vi "Multicolumn listbox Helper.vi"(4 "Row to Delete":i32, 5 "Sheet Colors":T1, 6 "Visible rows":i32=16, 7 "Multicolumn Ref":refnum<vi>, 8 "Error In":errorcluster, 9 "2D Data":string[][](array[string]), 10 "Data":string[](array[string]), 11 "Action (add default)":T2=enum."Add") -> (0 "Error Out":errorcluster)   [LabVIEW 2012]
doc: "The .vi is used with a \"Multicolumn Listbox\" \n\nHow to use.\nInit:\n1.Reference to Multicolumn Listbox (this is a functional global so you only need to set it once)\n2.Set action to Init\n3.Set names on columns, last column (Status) will be added automatic (Init also sets the nummber of visible columns)\n4.Set nummber of visible rows (if you add more data then visible rows the vertical scrollbar will be visible)\n5.Colors (optional) use if you want to change colors for OK, FAIL and clear (this is a functional global so you only need to set it once)\n\nClear:\nJust set Action to Clear, no other inputs needed\n\nAdd:\nTo Add data to the listbox you need to use two inputs\n1. Status sets the color of the row and OK or FAIL in the last column (Status)\n2. Data Is an array of strings, one string for each column you have defined in Init\n3.Action Add is default so it is not necessary to set\nIf you add more lines then set in init the vertical scrollbar will be visible"
uses:
  Controls/Spreadsheet Commands.ctl
  Controls/Sheet Colors.ctl
  <vilib>/Utility/miscctls.llb/LVRowAndColumnTypeDef.ctl
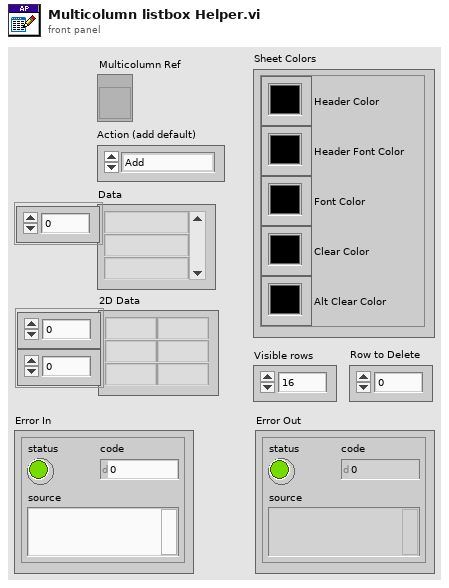
[diagram p1: front panel]
types:
  T1 = typedef "Sheet Colors.ctl" = cluster{"Header Color":u32, "Header Font Color":u32, "Font Color":u32, "Clear Color":u32, "Alt Clear Color":u32}
  T2 = typedef "Spreadsheet Commands.ctl" = enum16{"Init", "Clear", "Add", "Mass Add", "Delete Row", "Format Colors"}
  T3 = typedef "LVRowAndColumnTypeDef.ctl" = cluster{"Row":i32, "Column":i32}
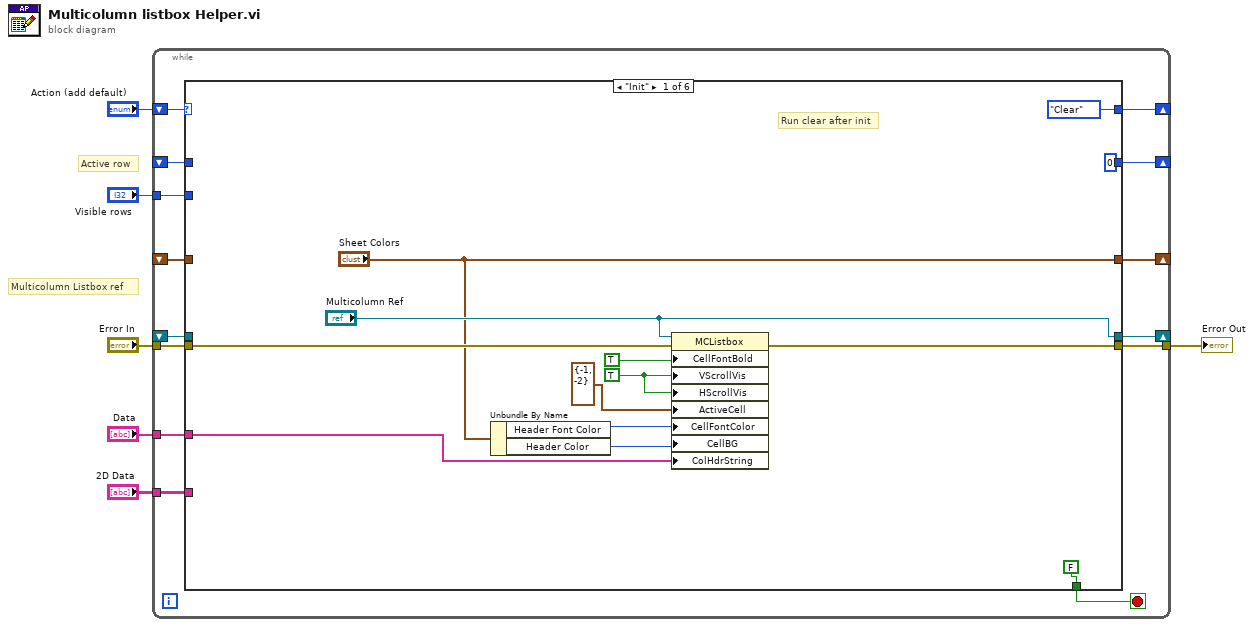
[diagram p0: block diagram]
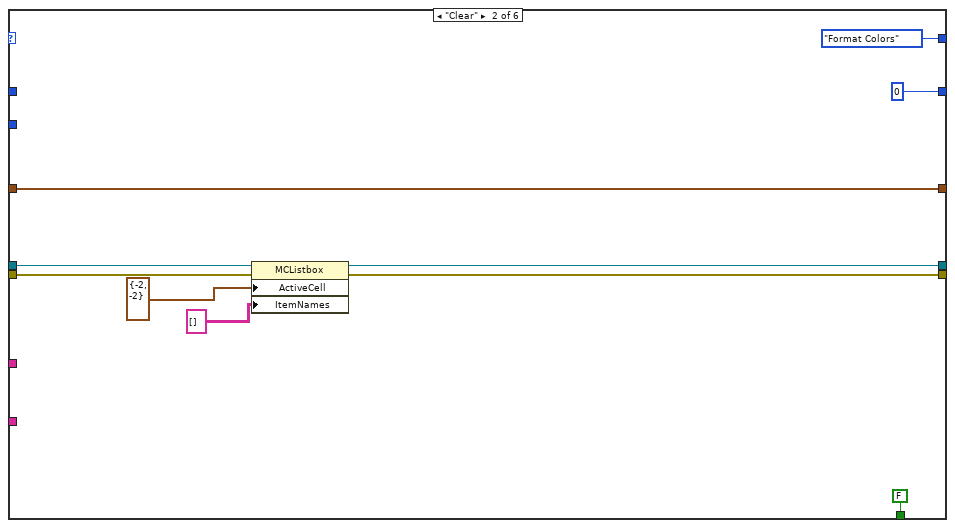
[diagram p2: hidden frame]
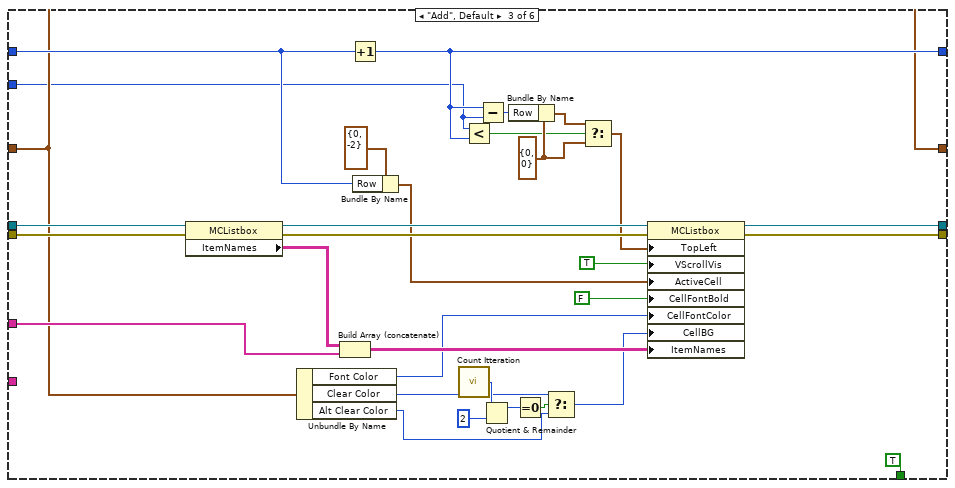
[diagram p3: hidden frame]
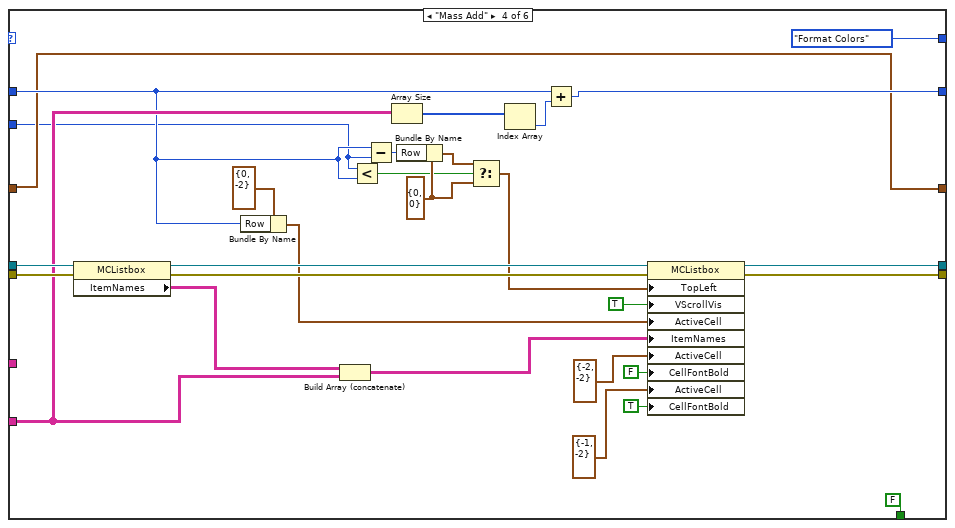
[diagram p4: hidden frame]
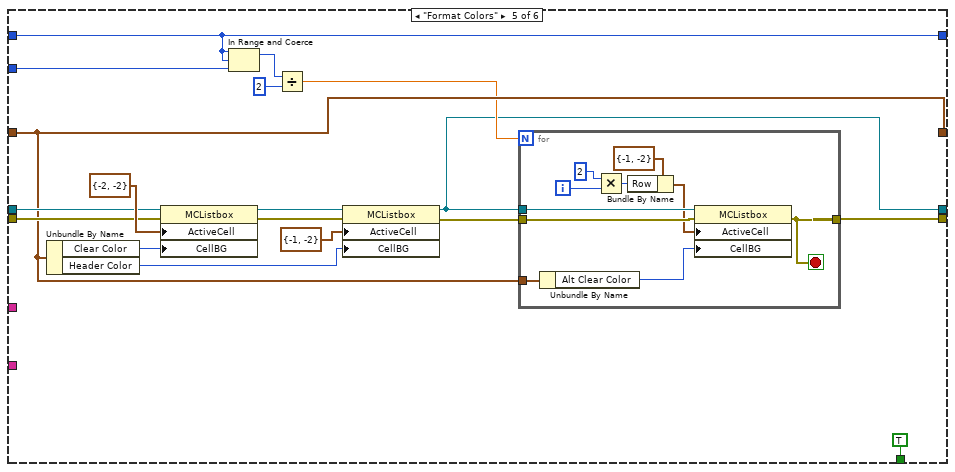
[diagram p5: hidden frame]
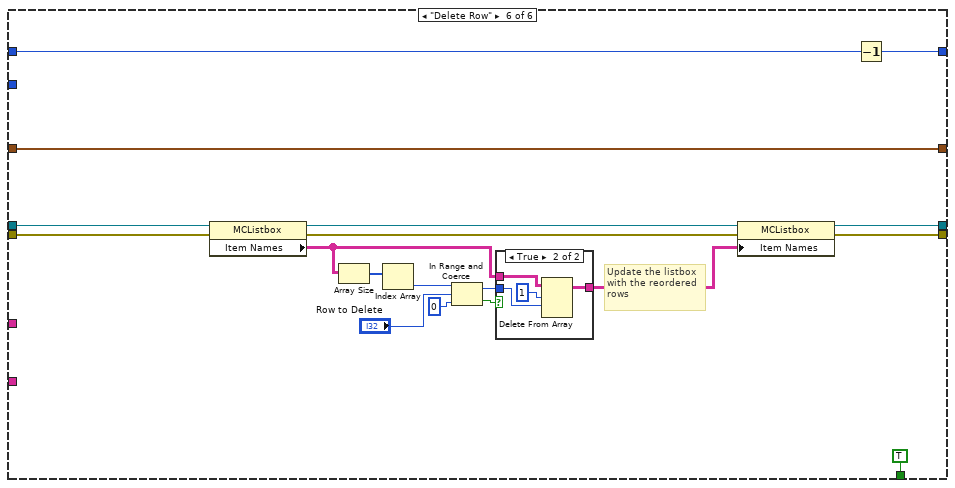
[diagram p6: hidden frame]
diagram:
  # "Active row"
  # "Multicolumn Listbox ref"
  n1 = while {
    shift-right: [w19] -> _
    shift-left: _ -> [w20]
    tunnel: "Error In" -> [w18]
    tunnel: [w17] -> w5
    shift-right: [w15] -> _
    shift-left: "Action (add default)" -> [w16]
    shift-right: [w13] -> _
    shift-left: _ -> [w12]
    tunnel: "Visible rows" -> [w11]
    tunnel: "Data" -> [w10]
    tunnel: "2D Data" -> [w9]
    shift-right: [w8] -> _
    shift-left: _ -> [w7]
    stop <- w14 stop-if-true
    n2 = case shown="\"Init\"" w16 {
      tunnel: w20 -> [_ w42 w67 w96 w118 w139]
      tunnel: ["Multicolumn Ref" w36 w63 w81 w104 w137] -> w19
      tunnel: w18 -> [w25 w41 w66 w95 w117 w140]
      tunnel: [w27 w35 w62 w93 w106 w138] -> w17
      tunnel: [Spreadsheet_Commands."Clear" ("Action (add default)") Spreadsheet_Commands."Format Colors" ("Action (add default)") _ Spreadsheet_Commands."Format Colors" ("Action (add default)") _ _] -> w15
      tunnel: [FALSE FALSE TRUE FALSE TRUE TRUE] -> w14
      tunnel: [0 ("Row") 0 ("Row") w57 w90 w108 w135] -> w13
      tunnel: w12 -> [_ _ w64 w82 w108 w136]
      tunnel: w11 -> [_ _ w44 w75 w109 _]
      tunnel: w10 -> [w26 _ w55 _ _ _]
      tunnel: w9 -> [_ _ _ w88 _ _]
      tunnel: w7 -> [_ w34 w48 w76 w110 w133]
      tunnel: ["Sheet Colors" w34 w48 w76 w110 w133] -> w8
      frame "Init" {
        w32 = TRUE
        # "Run clear after init"
        n3 = Unbundle By Name("Sheet Colors") -> ("Header Font Color"=w23:u32, "Header Color"=w24:u32)
        n4 = property class="MCListbox"(reference="Multicolumn Ref", error in=w25, "CellFontBold"=TRUE ("Active Cell:Cell Font:Bold"), "VScrollVis"=w32, "HScrollVis"=w32, "ActiveCell"=T3 {"Row"=-1, "Column"=-2} ("Active Cell:Active Cell"), "CellFontColor"=w23, "CellBG"=w24, "ColHdrString"=w26) -> (error out=w27:errorcluster)  [unwired: 1 out]
      }
      frame "Clear" {
        n5 = property class="MCListbox"(reference=w42, error in=w41, "ActiveCell"=T3 {"Row"=-2, "Column"=-2} ("Active Cell:Active Cell"), "ItemNames"=string[][] []) -> (reference out=w36:refnum<vi>, error out=w35:errorcluster)
      }
      frame "Add", Default {
        w70 = T3 {"Row"=0, "Column"=0} ("Active Cell:Active Cell")
        n6 = property class="MCListbox"(reference=w67, error in=w66) -> (reference out=w74:refnum<vi>, error out=w71:errorcluster, "ItemNames"=w60:string[][])
        n7 = Unbundle By Name(w48) -> ("Font Color"=w47:u32, "Clear Color"=w46:u32, "Alt Clear Color"=w45:u32)
        n8 = Build Array (concatenate)(w60, w55) -> (w58:string[][])
        n9 = Increment(x=w64) -> (x+1=w57:i32)
        n10 = Bundle By Name(cluster=T3 {"Row"=0, "Column"=-2} ("Active Cell:Active Cell"), "Row"=w64) -> (w61:T3)
        n11 = call "Count Itteration.vi"() -> ("Itteration"=w54:i32)  [unwired: 7 in, 1 out]
        n12 = Less?(x=w44, y=w57) -> (x < y?=w56:bool)
        n13 = Subtract(x=w57, y=w44) -> (x-y=w73:i32)
        n14 = Quotient & Remainder(x=w54, y=2) -> (x-y*floor(x/y)=w52:i32)  [unwired: 1 out]
        n15 = Bundle By Name(cluster=w70, "Row"=w73) -> (w72:T3)
        n16 = Equal To 0?(x=w52) -> (x = 0?=w51:bool)
        n17 = Select(t=w46, s=w51, f=w45) -> (s? t:f=w50:u32)
        n18 = Select(t=w72, s=w56, f=w70) -> (s? t:f=w69:T3)
        n19 = property class="MCListbox"(reference=w74, error in=w71, "TopLeft"=w69, "VScrollVis"=TRUE ("Visible Items:Vertical Scrollbar Visible"), "ActiveCell"=w61, "CellFontBold"=FALSE ("Caption.Font:Bold"), "CellFontColor"=w47, "CellBG"=w50, "ItemNames"=w58) -> (reference out=w63:refnum<vi>, error out=w62:errorcluster)
      }
      frame "Mass Add" {
        w99 = T3 {"Row"=0, "Column"=0} ("Active Cell:Active Cell")
        n20 = property class="MCListbox"(reference=w96, error in=w95) -> (reference out=w103:refnum<vi>, error out=w100:errorcluster, "ItemNames"=w91:string[][])
        n21 = Bundle By Name(cluster=T3 {"Row"=0, "Column"=-2} ("Active Cell:Active Cell"), "Row"=w82) -> (w92:T3)
        n22 = Build Array (concatenate)(w91, w88) -> (w84:string[][])
        n23 = Less?(x=w75, y=w82) -> (x < y?=w89:bool)
        n24 = Subtract(x=w82, y=w75) -> (x-y=w102:i32)
        n25 = Array Size(array=w88) -> (size(s)=w87:i32[])
        n26 = Bundle By Name(cluster=w99, "Row"=w102) -> (w101:T3)
        n27 = Select(t=w101, s=w89, f=w99) -> (s? t:f=w98:T3)
        n28 = Index Array(array=w87) -> (element=w86:i32)  [unwired: 1 in]
        n29 = Add(x=w82, y=w86) -> (x+y=w90:i32)
        n30 = property class="MCListbox"(reference=w103, error in=w100, "TopLeft"=w98, "VScrollVis"=TRUE ("Visible Items:Vertical Scrollbar Visible"), "ActiveCell"=w92, "ItemNames"=w84, "ActiveCell"=T3 {"Row"=-2, "Column"=-2} ("Active Cell:Active Cell"), "CellFontBold"=FALSE ("Active Cell:Cell Font:Bold"), "ActiveCell"=T3 {"Row"=-1, "Column"=-2} ("Active Cell:Active Cell"), "CellFontBold"=TRUE ("Active Cell:Cell Font:Bold")) -> (reference out=w81:refnum<vi>, error out=w93:errorcluster)
      }
      frame "Format Colors" {
        n31 = Unbundle By Name(w110) -> ("Clear Color"=w113:u32, "Header Color"=w111:u32)
        n32 = property class="MCListbox"(reference=w118, error in=w117, "ActiveCell"=T3 {"Row"=-2, "Column"=-2} ("Active Cell:Active Cell"), "CellBG"=w113) -> (reference out=w116:refnum<vi>, error out=w115:errorcluster)
        n33 = In Range and Coerce(upper limit=w108, x=w108, lower limit=w109) -> (coerced(x)=w107:i32)  [unwired: 1 out]
        n34 = Divide(x=w107, y=2) -> (x/y=w105:dbl)
        n35 = property class="MCListbox"(reference=w116, error in=w115, "ActiveCell"=T3 {"Row"=-1, "Column"=-2} ("Active Cell:Active Cell"), "CellBG"=w111) -> (reference out=w104:refnum<vi>, error out=w114:errorcluster)
        n36 = for {
          N: w105 -> [_]
          tunnel: w104 -> [w128]
          tunnel: w114 -> [w127]
          tunnel: w110 -> [w125]
          tunnel: [w123] -> w106
          i -> [w130]
          stop <- w123 stop-if-true
          n37 = Unbundle By Name(w125) -> ("Alt Clear Color"=w126:u32)
          n38 = Multiply(x=2, y=w130) -> (x*y=w122:i32)
          n39 = Bundle By Name(cluster=T3 {"Row"=-1, "Column"=-2} ("Active Cell:Active Cell"), "Row"=w122) -> (w124:T3)
          n40 = property class="MCListbox"(reference=w128, error in=w127, "ActiveCell"=w124, "CellBG"=w126) -> (error out=w123:errorcluster)  [unwired: 1 out]
        }
      }
      frame "Delete Row" {
        # "Update the listbox\nwith the reordered\nrows"
        n41 = property class="MCListbox"(reference=w139, error in=w140) -> (reference out=w147:refnum<vi>, error out=w148:errorcluster, "Item Names"=w146:string[][])
        n42 = Array Size(array=w146) -> (size(s)=w145:i32[])
        n43 = Index Array(array=w145) -> (element=w144:i32)  [unwired: 1 in]
        n44 = In Range and Coerce(upper limit=w144, x="Row to Delete", lower limit=0) -> (coerced(x)=w142:i32, In Range?=w141:bool)
        n45 = case shown="True" w141 {
          tunnel: w146 -> [w150 w154]
          tunnel: [w150 w153] -> w149
          tunnel: w142 -> [_ w151]
          frame False {
          }
          frame True {
            n46 = Delete From Array(array=w154, length=1, index (row)=w151) -> (array with subset deleted=w153:string[][])  [unwired: 1 in, 1 out]
          }
        }
        n47 = property class="MCListbox"(reference=w147, error in=w148, "Item Names"=w149) -> (reference out=w137:refnum<vi>, error out=w138:errorcluster)
        n48 = Decrement(x=w136) -> (x-1=w135:i32)
      }
    }
  }
  "Error Out" <- w5
